vi "CmdBuilder.vi"(9 "ChatId":i32, 11 "InText":string) -> (3 "Cmd":T2={"Cmd"=["Default", "/getweather", "/led1", "/led2", "/led3", "/gettime", "on", "off", "delete keyboard", "/start"], "Param"=[], "CmdText"="", "ChatId"=0})   [LabVIEW 2015]
uses:
  Telegram/Methods/TypeDefs/CommandList.ctl
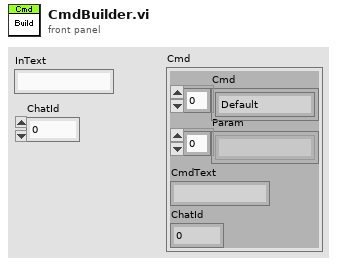
[diagram p1: front panel]
types:
  T1 = typedef "CommandList.ctl" = string[]
  T2 = cluster{"Cmd":T1, "Param":string[], "CmdText":string, "ChatId":i32}
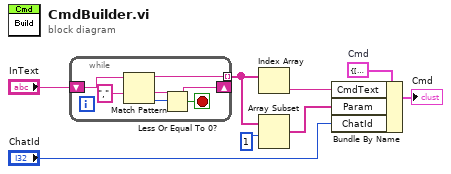
[diagram p0: block diagram]
diagram:
  w6 = T2 {"Cmd"=["Default", "/getweather", "/led1", "/led2", "/led3", "/gettime", "on", "off", "delete keyboard", "/start"], "Param"=[], "CmdText"="Default", "ChatId"=0}  # Cmd
  n1 = while {
    shift-right: [w12] -> _
    shift-left: "InText" -> [w13]
    tunnel: [w11] -> w8 mode=indexing
    stop <- w10 stop-if-true
    n2 = Match Pattern(string=w13, regular expression=",") -> (before substring=w11:string, after substring=w12:string, offset past match=w9:i32)  [unwired: 1 in, 1 out]
    n3 = Less Or Equal To 0?(x=w9) -> (x <= 0?=w10:bool)
  }
  n4 = Index Array(array=w8) -> (element=w1:string)  [unwired: 1 in]
  n5 = Array Subset(array=w8, index=1) -> (w2:string[])  [unwired: 1 in]
  n6 = Bundle By Name(cluster=w6, "CmdText"=w1, "Param"=w2, "ChatId"="ChatId") -> (→"Cmd":T2)
